vi "Jog.vi"(0 "MG17Motor":refnum<k7>(container), 1 "error in (no error)":errorcluster, 2 "Current Pos":refnum<vi>, 3 "Complete?":refnum<vi>, 4 "Stop":refnum<vi>) -> (5 "reference out":refnum<k7>, 6 "error out":errorcluster)   [LabVIEW 2010]
panel:
  out "Current":dbl
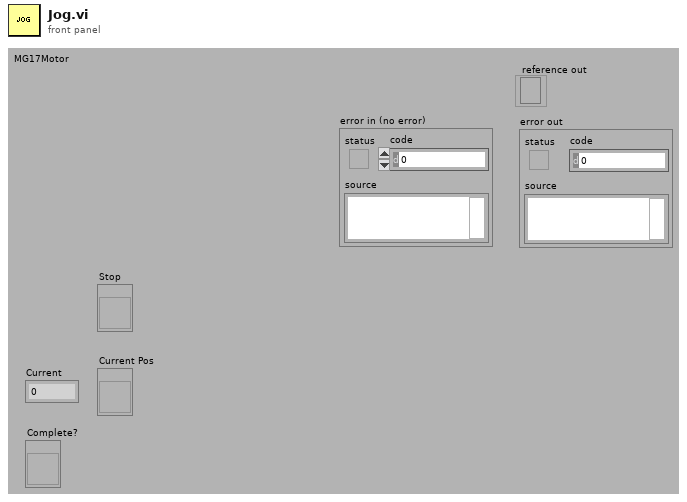
[diagram p1: front panel]
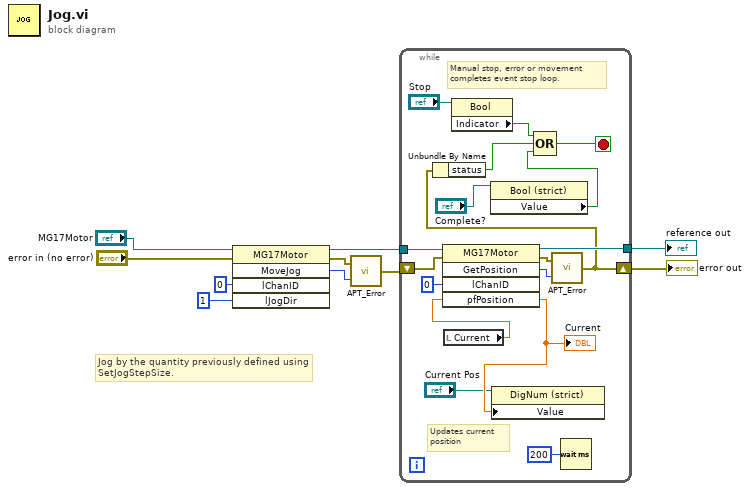
[diagram p0: block diagram]
diagram:
  # "Jog by the quantity previously defined using\nSetJogStepSize."
  n1 = invoke class="MG17Motor" method="MoveJog"(reference="MG17Motor", error in="error in (no error)", "lChanID"=0, "lJogDir"=1) -> (reference out=w6:refnum<k7>, error out=w9:errorcluster, "MoveJog"=w8:i32)  [unwired: 1 in, 2 out]
  n2 = call "APT_Error.vi"("Return Code"=w8, "error in (no error)"=w9) -> ("error out"=w7:errorcluster)
  n3 = while {
    shift-right: [w20] -> w5
    shift-left: w7 -> [w23]
    tunnel: w6 -> [w25]
    tunnel: [w24] -> w4
    stop <- w18 stop-if-true
    # "Updates current\nposition"
    # "Manual stop, error or movement\ncompletes event stop loop."
    n4 = local read "Current"() -> (w16:dbl)
    n5 = invoke class="MG17Motor" method="GetPosition"(reference=w25, error in=w23, "lChanID"=0, "pfPosition"=w16) -> (reference out=w24:refnum<k7>, error out=w27:errorcluster, "GetPosition"=w26:i32, "pfPosition"=w17:sgl)  [unwired: 1 in, 1 out]
    "Current" <- w17
    n6 = property class="Bool"(reference="Stop") -> ("Indicator"=w11:bool)  [unwired: 1 in, 2 out]
    n7 = property class="Bool (strict)"(reference="Complete?") -> ("Value"=w13:bool)  [unwired: 1 in, 2 out]
    n8 = property class="DigNum (strict)"(reference="Current Pos", "Value"=w17) -> ()  [unwired: 1 in, 2 out]
    n9 = call "APT_Error.vi"("Return Code"=w26, "error in (no error)"=w27) -> ("error out"=w20:errorcluster)
    n10 = Unbundle By Name(w20) -> ("status"=w19:bool)
    n11 = Compound Arithmetic op=OR(w11, w19, w13) -> (w18:bool)
    n12 = Wait (ms)(milliseconds to wait=u32 200) -> ()  [unwired: 1 out]
  }
  "reference out" <- w4
  "error out" <- w5
